vi "Prueba_MAIN.vi"() -> ()   [LabVIEW 2019]
uses:
  Estados_flujo_Debug.ctl
  CLUSTER_CONTROLES_INDICADORES.ctl
  Acciones_UI.ctl
  <vilib>/Instr/_visa.llb/VISA Configure Serial Port (Instr).vi
panel:
  out "Numeric":i32
  in  "Tab Control":enum32{"Page 1", "Page 2"}(tab)
  out "MESSAGES":string
  in  "TEST ASICS":bool
  in  "MOVER ASICS":bool
  in  "LEER QR'S":bool
  in  "CALIBRACION":bool
  in  "Exit":bool
  in  "INICIAR COM":bool
  out "DISPOSITIVO CONECTADO":string
  # "PONER VENTANA DE DIALOGO PARA PREGUNTAR SI SE QUIERE SALIR CUANDO SE PRESIONE STOP"
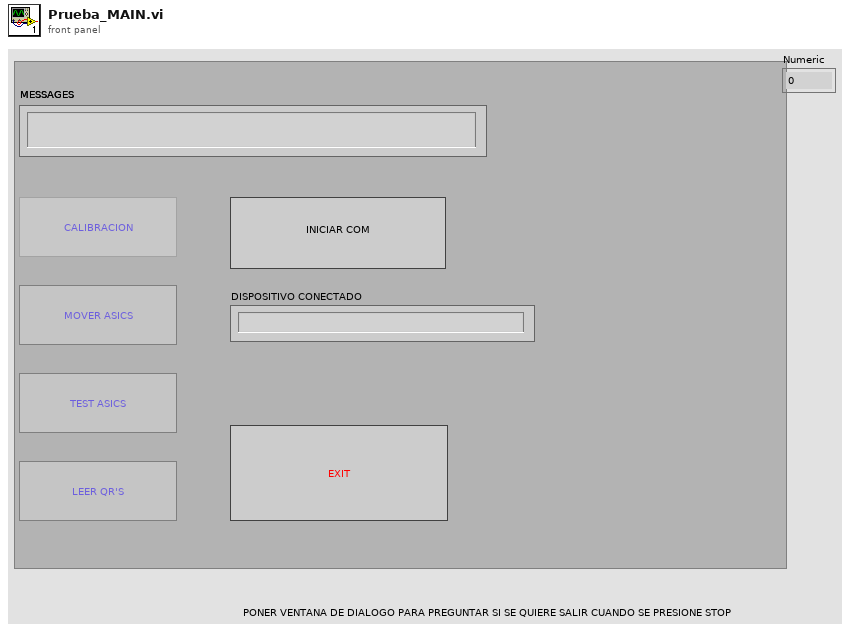
[diagram p1: front panel]
types:
  T1 = typedef "CLUSTER_CONTROLES_INDICADORES.ctl" = cluster{"TEST ASICS":refnum<vi>, "MOVER ASICS":refnum<vi>, "LEER QR'S":refnum<vi>, "MESSAGES":refnum<vi>, "INICIAR COM":refnum<vi>, "stop":refnum<vi>, "CALIBRACION":refnum<vi>}
  T2 = typedef "Estados_flujo_Debug.ctl" = enum16{"Init", "Sesiones Visa abiertas?", "Iniciar Visa", "Start", "Enviar Comando", "Recibir Fin", "Error?"}
  T3 = typedef "Acciones_UI.ctl" = enum16{"Activar", "Desactivar", "Reiniciar default"}
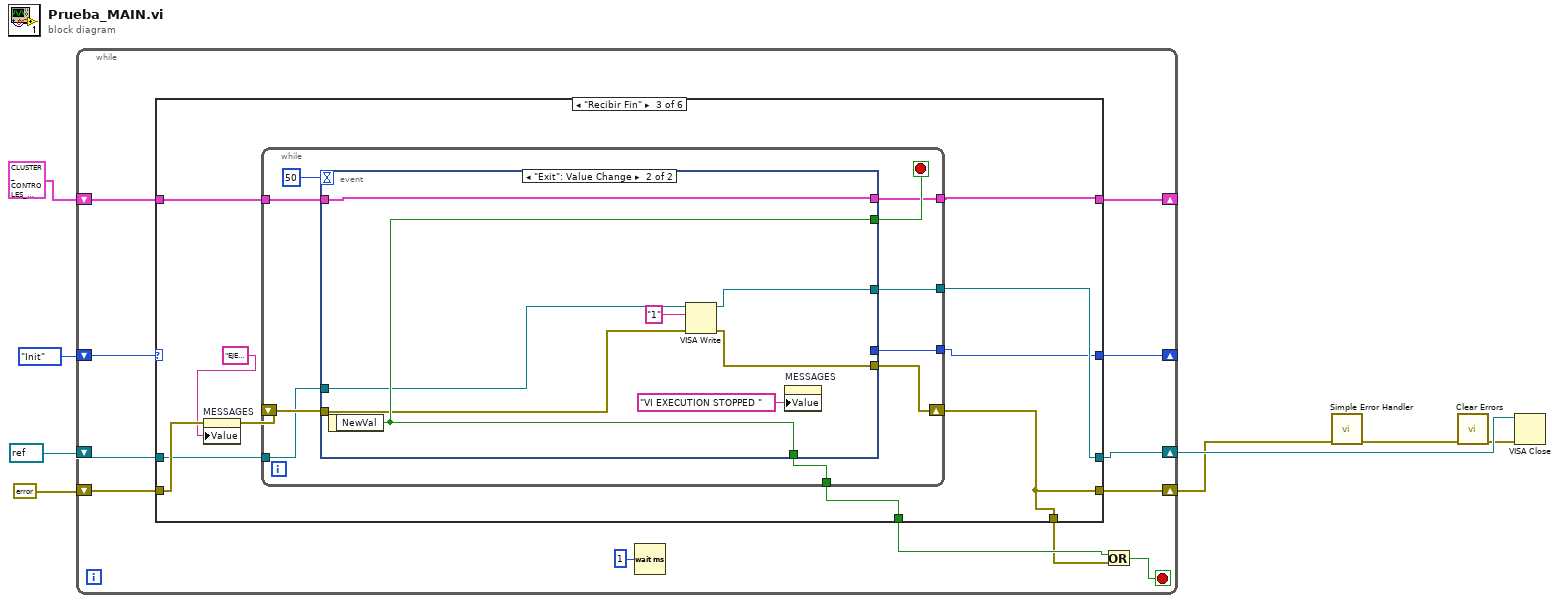
[diagram p0: block diagram]
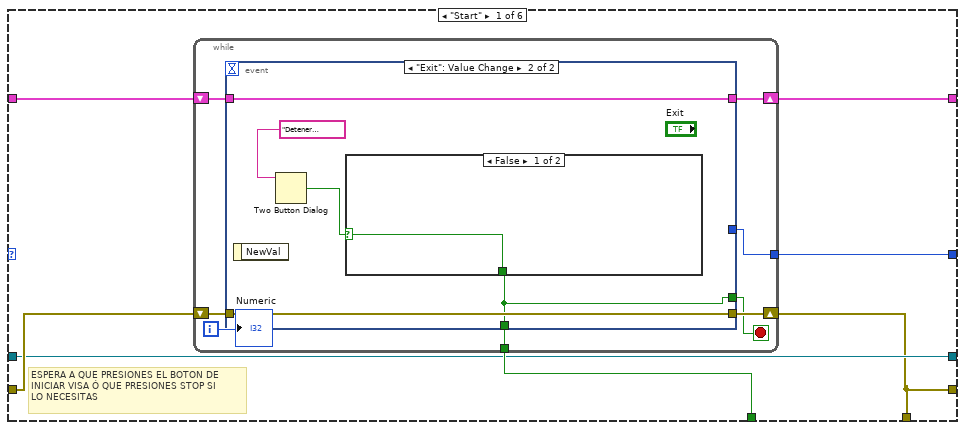
[diagram p2: hidden frame]
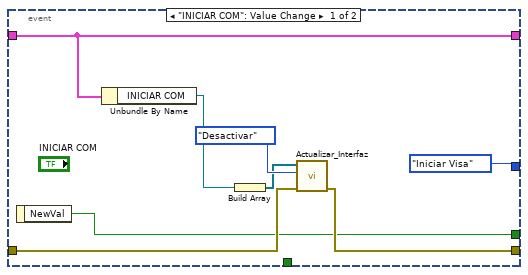
[diagram p3: hidden frame]
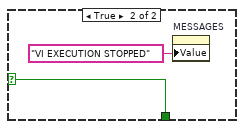
[diagram p4: hidden frame]
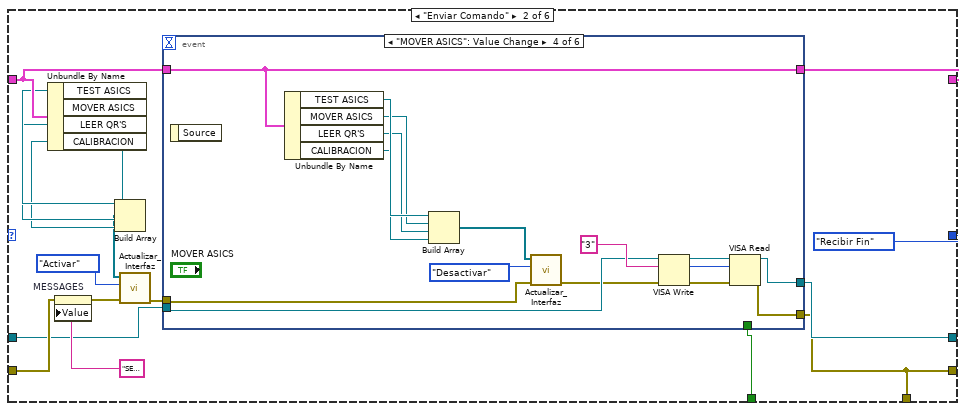
[diagram p5: hidden frame]
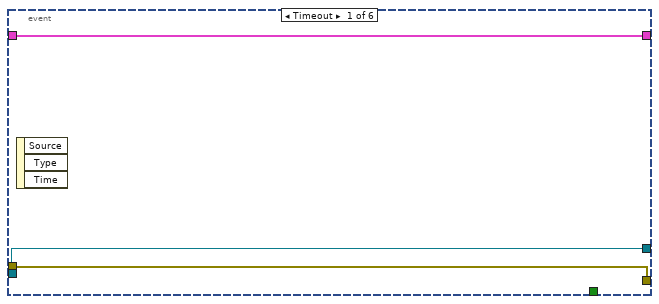
[diagram p6: hidden frame]
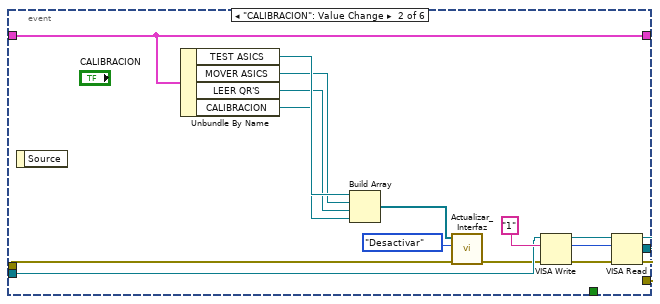
[diagram p7: hidden frame]
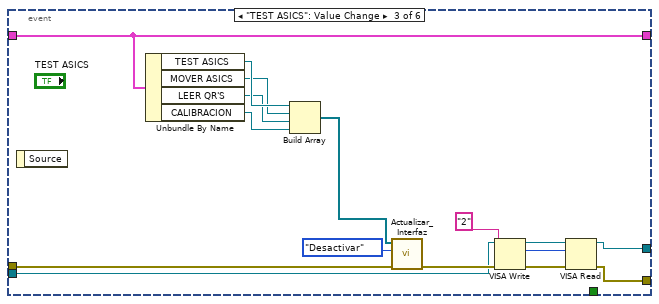
[diagram p8: hidden frame]
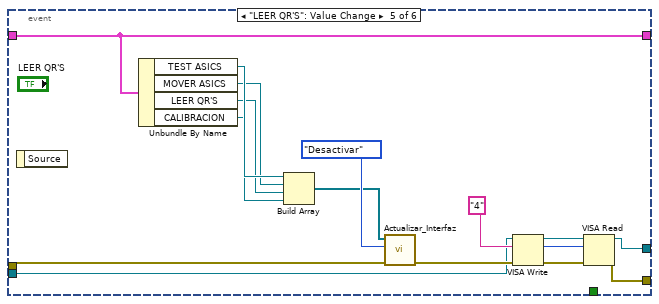
[diagram p9: hidden frame]
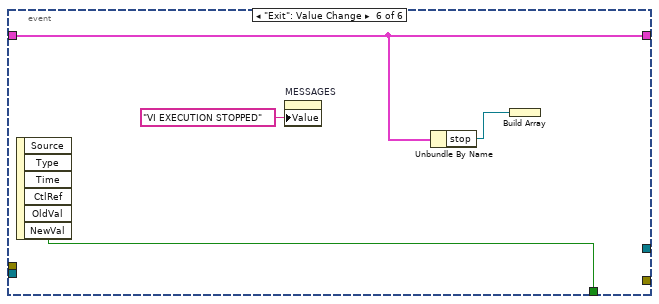
[diagram p10: hidden frame]
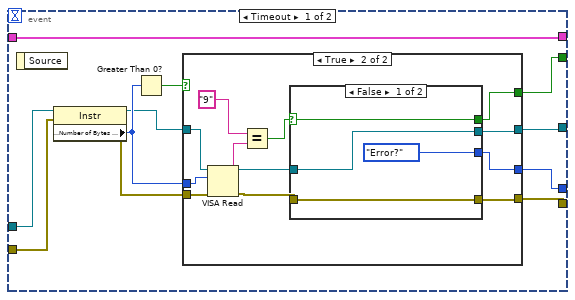
[diagram p11: hidden frame]
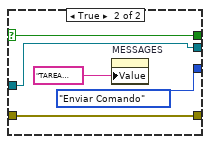
[diagram p13: hidden frame]
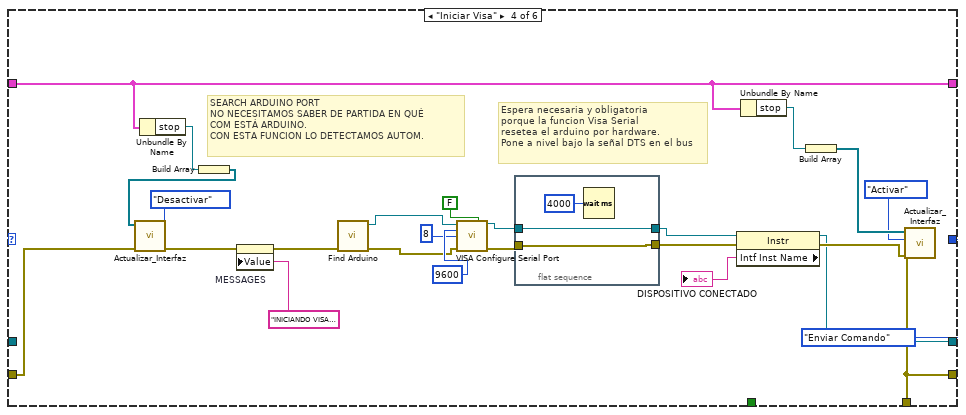
[diagram p14: hidden frame]
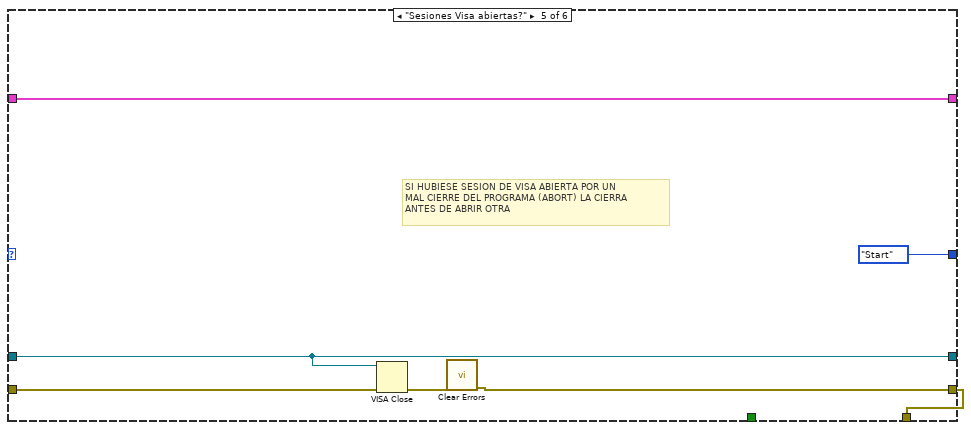
[diagram p15: hidden frame]
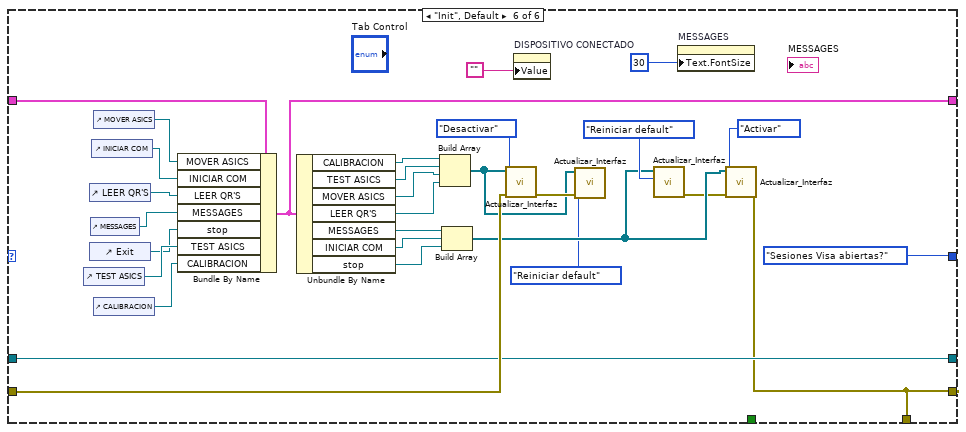
[diagram p16: hidden frame]
diagram:
  n1 = while {
    shift-right: [w17] -> _
    shift-left: Estados_flujo_Debug."Init" -> [w20]
    shift-right: [w16] -> w2
    shift-left: errorcluster {"status"=FALSE, "code"=0, "source"=""} ("error out") -> [w18]
    shift-right: [w10] -> w6
    shift-left: refnum<visa-resource-name> refnum ("VISA resource name out") -> [w11]
    shift-right: [w12] -> _
    shift-left: T1 {"TEST ASICS"=refnum, "MOVER ASICS"=refnum, "LEER QR'S"=refnum, "MESSAGES"=refnum, "INICIAR COM"=refnum, "stop"=refnum, "CALIBRACION"=refnum} ("INDICADORES_CONTROLES") -> [w13]
    stop <- w15 stop-if-true
    n2 = case shown="\"Recibir Fin\"" w20 {
      tunnel: [w27 w68 w143 _ _ _] -> w19
      tunnel: w18 -> [w24 w63 w147 w215 w234 w247]
      tunnel: [w22 w52 w139 w206 w230 w240] -> w16
      tunnel: [w21 Estados_flujo_Debug."Recibir Fin" w138 Estados_flujo_Debug."Enviar Comando" Estados_flujo_Debug."Start" ("f") Estados_flujo_Debug."Sesiones Visa abiertas?"] -> w17
      tunnel: [w23 w65 w144 w201 w231 w245] -> w10
      tunnel: w13 -> [w26 w60 w141 w207 w232 w246]
      tunnel: [w25 w64 w140 w207 w232 w244] -> w12
      tunnel: w11 -> [w23 w62 w142 _ w231 w245]
      tunnel: [w22 w52 w139 w206 w230 w240] -> w9
      frame "Start" {
        # "ESPERA A QUE PRESIONES EL BOTON DE\nINICIAR VISA Ó QUE PRESIONES STOP SI\nLO NECESITAS"
        n3 = while {
          tunnel: [w35] -> w27
          tunnel: [w30] -> w21
          shift-right: [w33] -> w25
          shift-left: w26 -> [w34]
          shift-right: [w31] -> w22
          shift-left: w24 -> [w32]
          i -> [w28]
          stop <- w29 stop-if-true
          n4 = event shown="[1] \"Exit\": Value Change" {
            selector: _ -> [_ _]
            dyn-events: _ -> [_ _]
            timeout: _ -> [_ _]
            tunnel: [_ w44] -> w35
            tunnel: [Estados_flujo_Debug."Iniciar Visa" ("f") _] -> w30
            tunnel: w32 -> [w38 w48]
            tunnel: [w37 w48] -> w31
            tunnel: w34 -> [w41 w46]
            tunnel: [w41 w46] -> w33
            tunnel: [w36 w44] -> w29
            event "INICIAR COM": Value Change {
              n5 = event-data() -> ("NewVal"=w36:bool)  [unwired: 1 in]
              n6 = Unbundle By Name(w41) -> ("INICIAR COM"=w40:refnum<vi>)
              n7 = Build Array(w40) -> (w39:refnum<vi>[])
              n8 = call "Actualizar_Interfaz.vi"("error in (no error)"=w38, "Enum"=Acciones_UI."Desactivar", "Controls"=w39) -> ("error out"=w37:errorcluster)  [unwired: 8 in]
            }
            event "Exit": Value Change {
              n9 = event-data() -> ()  [unwired: 1 in, 1 out]
              n10 = Two Button Dialog(message="Detener ejecución?") -> (T button?=w47:bool)  [unwired: 2 in]
              n11 = case shown="False" w47 {
                selector: w47 -> [w49 w50]
                tunnel: [w49 w50] -> w44
                frame False {
                }
                frame True {
                  n12 = property on="MESSAGES" class="Str"("Value"="VI EXECUTION STOPPED" ("MESSAGES")) -> ()  [unwired: 2 in, 2 out]
                }
              }
            }
          }
          "Numeric" <- w28
        }
      }
      frame "Enviar Comando" {
        n13 = Unbundle By Name(w60) -> ("TEST ASICS"=w59:refnum<vi>, "MOVER ASICS"=w58:refnum<vi>, "LEER QR'S"=w57:refnum<vi>, "CALIBRACION"=w56:refnum<vi>)
        n14 = property on="MESSAGES" class="Str"(error in=w63, "Value"="SELECCIONE TAREA" ("String")) -> (error out=w61:errorcluster)  [unwired: 1 in, 1 out]
        n15 = Build Array(w59, w58, w57, w56) -> (w55:refnum<vi>[])
        n16 = call "Actualizar_Interfaz.vi"("error in (no error)"=w61, "Enum"=Acciones_UI."Activar", "Controls"=w55) -> ("error out"=w66:errorcluster)  [unwired: 8 in]
        n17 = event shown="[3] \"MOVER ASICS\": Value Change" {
          selector: _ -> [_ _ _ _ _ _]
          dyn-events: _ -> [_ _ _ _ _ _]
          timeout: _ -> [_ _ _ _ _ _]
          tunnel: [_ _ _ _ _ w137] -> w68
          tunnel: w66 -> [w69 w73 w95 w104 w127 _]
          tunnel: [w70 w85 w97 w105 w129 _] -> w65
          tunnel: [w69 w84 w98 w114 w128 _] -> w52
          tunnel: w60 -> [w71 w74 w96 w106 w119 w134]
          tunnel: [w71 w74 w96 w106 w119 w134] -> w64
          tunnel: w62 -> [w70 w81 w94 w113 w126 _]
          event Timeout {
            n18 = event-data() -> ()  [unwired: 1 in, 3 out]
          }
          event "CALIBRACION": Value Change {
            n19 = event-data() -> ()  [unwired: 1 in, 1 out]
            n20 = Unbundle By Name(w74) -> ("TEST ASICS"=w80:refnum<vi>, "MOVER ASICS"=w79:refnum<vi>, "LEER QR'S"=w78:refnum<vi>, "CALIBRACION"=w77:refnum<vi>)
            n21 = Build Array(w80, w79, w78, w77) -> (w75:refnum<vi>[])
            n22 = call "Actualizar_Interfaz.vi"("error in (no error)"=w73, "Enum"=Acciones_UI."Desactivar", "Controls"=w75) -> ("error out"=w72:errorcluster)  [unwired: 8 in]
            n23 = VISA Write(VISA resource name=w81, write buffer="1", error in (no error)=w72) -> (VISA resource name out=w86:refnum<visa-resource-name>, return count=w82:u32, error out=w87:errorcluster)
            n24 = VISA Read(VISA resource name=w86, byte count=w82, error in (no error)=w87) -> (VISA resource name out=w85:refnum<visa-resource-name>, error out=w84:errorcluster)  [unwired: 2 out]
          }
          event "TEST ASICS": Value Change {
            n25 = event-data() -> ()  [unwired: 1 in, 1 out]
            n26 = Unbundle By Name(w96) -> ("TEST ASICS"=w93:refnum<vi>, "MOVER ASICS"=w92:refnum<vi>, "LEER QR'S"=w91:refnum<vi>, "CALIBRACION"=w90:refnum<vi>)
            n27 = Build Array(w93, w92, w91, w90) -> (w88:refnum<vi>[])
            n28 = call "Actualizar_Interfaz.vi"("Enum"=Acciones_UI."Desactivar", "Controls"=w88) -> ()  [unwired: 9 in, 1 out]
            n29 = VISA Write(VISA resource name=w94, write buffer="2", error in (no error)=w95) -> (VISA resource name out=w101:refnum<visa-resource-name>, return count=w99:u32, error out=w102:errorcluster)
            n30 = VISA Read(VISA resource name=w101, byte count=w99, error in (no error)=w102) -> (VISA resource name out=w97:refnum<visa-resource-name>, error out=w98:errorcluster)  [unwired: 2 out]
          }
          event "MOVER ASICS": Value Change {
            n31 = event-data() -> ()  [unwired: 1 in, 1 out]
            n32 = Unbundle By Name(w106) -> ("TEST ASICS"=w112:refnum<vi>, "MOVER ASICS"=w111:refnum<vi>, "LEER QR'S"=w110:refnum<vi>, "CALIBRACION"=w109:refnum<vi>)
            n33 = Build Array(w112, w111, w110, w109) -> (w107:refnum<vi>[])
            n34 = call "Actualizar_Interfaz.vi"("error in (no error)"=w104, "Enum"=Acciones_UI."Desactivar", "Controls"=w107) -> ("error out"=w103:errorcluster)  [unwired: 8 in]
            n35 = VISA Write(VISA resource name=w113, write buffer="3", error in (no error)=w103) -> (VISA resource name out=w117:refnum<visa-resource-name>, return count=w115:u32, error out=w118:errorcluster)
            n36 = VISA Read(VISA resource name=w117, byte count=w115, error in (no error)=w118) -> (VISA resource name out=w105:refnum<visa-resource-name>, error out=w114:errorcluster)  [unwired: 2 out]
          }
          event "LEER QR'S": Value Change {
            n37 = event-data() -> ()  [unwired: 1 in, 1 out]
            n38 = Unbundle By Name(w119) -> ("TEST ASICS"=w125:refnum<vi>, "MOVER ASICS"=w124:refnum<vi>, "LEER QR'S"=w123:refnum<vi>, "CALIBRACION"=w122:refnum<vi>)
            n39 = Build Array(w125, w124, w123, w122) -> (w120:refnum<vi>[])
            n40 = call "Actualizar_Interfaz.vi"("Enum"=Acciones_UI."Desactivar", "Controls"=w120) -> ()  [unwired: 9 in, 1 out]
            n41 = VISA Write(VISA resource name=w126, write buffer="4", error in (no error)=w127) -> (VISA resource name out=w132:refnum<visa-resource-name>, return count=w130:u32, error out=w133:errorcluster)
            n42 = VISA Read(VISA resource name=w132, byte count=w130, error in (no error)=w133) -> (VISA resource name out=w129:refnum<visa-resource-name>, error out=w128:errorcluster)  [unwired: 2 out]
          }
          event "Exit": Value Change {
            n43 = event-data() -> ("NewVal"=w137:bool)  [unwired: 1 in, 5 out]
            n44 = property on="MESSAGES" class="Str"("Value"="VI EXECUTION STOPPED" ("MESSAGES")) -> ()  [unwired: 2 in, 2 out]
            n45 = Unbundle By Name(w134) -> ("stop"=w135:refnum<vi>)
            n46 = Build Array(w135) -> ()  [unwired: 1 out]
          }
        }
      }
      frame "Recibir Fin" {
        n47 = property on="MESSAGES" class="Str"(error in=w147, "Value"="EJECUTANDO TAREA" ("String")) -> (error out=w145:errorcluster)  [unwired: 1 in, 1 out]
        n48 = while {
          tunnel: [w155] -> w138
          tunnel: [w153] -> w144
          shift-right: [w152] -> w139
          shift-left: w145 -> [w154]
          tunnel: [w151] -> w143
          tunnel: w142 -> [w150]
          tunnel: w141 -> [w149]
          tunnel: [w148] -> w140
          stop <- w156 stop-if-true
          n49 = event shown="[1] \"Exit\": Value Change" {
            selector: _ -> [_ _]
            dyn-events: _ -> [_ _]
            timeout: 50 -> [_ _]
            tunnel: [w166 w200] -> w156
            tunnel: [w165 _] -> w155
            tunnel: w154 -> [w164 w198]
            tunnel: [w161 w197] -> w152
            tunnel: [w160 w195] -> w153
            tunnel: [_ w200] -> w151
            tunnel: w150 -> [w159 w194]
            tunnel: w149 -> [w158 w193]
            tunnel: [w158 w193] -> w148
            event Timeout {
              n50 = event-data() -> ()  [unwired: 1 in, 1 out]
              n51 = property class="Instr"(reference=w159, error in=w164) -> (reference out=w163:refnum<visa-resource-name>, error out=w162:errorcluster, "Serial Settings:Number of Bytes at Serial Port"=w167:u32)
              n52 = Greater Than 0?(x=w167) -> (x > 0?=w168:bool)
              n53 = case shown="True" w168 {
                selector: w168 -> [w171 _]
                tunnel: w167 -> [_ w183]
                tunnel: [w171 w177] -> w166
                tunnel: [_ w178] -> w165
                tunnel: w163 -> [w170 w180]
                tunnel: w162 -> [w169 w174]
                tunnel: [w169 w172] -> w161
                tunnel: [w170 w176] -> w160
                frame False {
                }
                frame True {
                  n54 = VISA Read(VISA resource name=w180, byte count=w183, error in (no error)=w174) -> (VISA resource name out=w175:refnum<visa-resource-name>, read buffer=w181:string, error out=w173:errorcluster)  [unwired: 1 out]
                  n55 = Equal?(x="9", y=w181) -> (x = y?=w179:bool)
                  n56 = case shown="False" w179 {
                    selector: w179 -> [w186 w190]
                    tunnel: [Estados_flujo_Debug."Error?" Estados_flujo_Debug."Enviar Comando"] -> w178
                    tunnel: [w186 w190] -> w177
                    tunnel: [w185 w189] -> w176
                    tunnel: w175 -> [w185 w189]
                    tunnel: w173 -> [w184 w188]
                    tunnel: [w184 w188] -> w172
                    frame False {
                    }
                    frame True {
                      n57 = property on="MESSAGES" class="Str"("Value"="TAREA TERMINADA" ("String")) -> ()  [unwired: 2 in, 2 out]
                    }
                  }
                }
              }
            }
            event "Exit": Value Change {
              n58 = event-data() -> ("NewVal"=w200:bool)  [unwired: 1 in]
              n59 = VISA Write(VISA resource name=w194, write buffer="1", error in (no error)=w198) -> (VISA resource name out=w195:refnum<visa-resource-name>, error out=w197:errorcluster)  [unwired: 1 out]
              n60 = property on="MESSAGES" class="Str"("Value"="VI EXECUTION STOPPED " ("MESSAGES")) -> ()  [unwired: 2 in, 2 out]
            }
          }
        }
      }
      frame "Iniciar Visa" {
        # "SEARCH ARDUINO PORT\nNO NECESITAMOS SABER DE PARTIDA EN QUÉ\nCOM ESTÁ ARDUINO. \nCON ESTA FUNCION LO DETECTAMOS AUTOM."
        # "Espera necesaria y obligatoria\nporque la funcion Visa Serial\nresetea el arduino por hardware.\nPone a nivel bajo la señal DTS en el bus"
        n61 = Unbundle By Name(w207) -> ("stop"=w213:refnum<vi>)
        n62 = Build Array(w213) -> (w212:refnum<vi>[])
        n63 = call "Actualizar_Interfaz.vi"("error in (no error)"=w215, "Enum"=Acciones_UI."Desactivar", "Controls"=w212) -> ("error out"=w214:errorcluster)  [unwired: 8 in]
        n64 = property on="MESSAGES" class="Str"(error in=w214, "Value"="INICIANDO VISA Y ARDUINO.....ESPERE" ("String")) -> (error out=w218:errorcluster)  [unwired: 1 in, 1 out]
        n65 = call "Find Arduino.vi"("error in (no error)"=w218) -> ("error out"=w223:errorcluster, "VISA resource name"=w222:refnum<visa-resource-name>)  [unwired: 8 in, 1 out]
        n66 = call-poly "VISA Configure Serial Port"("VISA resource name"=w222, "Enable Termination\nChar (T)"=FALSE ("Enable Termination\nChar (T)"), "baud rate (9600)"=u32 9600, "data bits (8)"=u16 8, "error in (no error)"=w223) -> ("VISA resource name out"=w203:refnum<visa-resource-name>, "error out"=w217:errorcluster)  [unwired: 9 in]
        n67 = flat-sequence {
          tunnel: [w227] -> w205
          tunnel: w217 -> [w227]
          tunnel: [w226] -> w202
          tunnel: w203 -> [w226]
          frame #0 {
            n68 = Wait (ms)(milliseconds to wait=u32 4000) -> ()  [unwired: 1 out]
          }
        }
        n69 = property class="Instr"(reference=w202, error in=w205) -> (reference out=w201:refnum<visa-resource-name>, error out=w204:errorcluster, "Intf Inst Name"=→"DISPOSITIVO CONECTADO":string)
        n70 = Unbundle By Name(w207) -> ("stop"=w210:refnum<vi>)
        n71 = Build Array(w210) -> (w209:refnum<vi>[])
        n72 = call "Actualizar_Interfaz.vi"("error in (no error)"=w204, "Enum"=Acciones_UI."Activar", "Controls"=w209) -> ("error out"=w206:errorcluster)  [unwired: 8 in]
      }
      frame "Sesiones Visa abiertas?" {
        # "SI HUBIESE SESION DE VISA ABIERTA POR UN \nMAL CIERRE DEL PROGRAMA (ABORT) LA CIERRA\nANTES DE ABRIR OTRA"
        n73 = VISA Close(VISA resource name=w231, error in (no error)=w234) -> (error out=w233:errorcluster)
        n74 = call <vilib>:"Clear Errors.vi"("error in (no error)"=w233) -> ("error out"=w230:errorcluster)  [unwired: 5 in, 1 out]
      }
      frame "Init", Default {
        n75 = control-ref of="TEST ASICS"() -> (w263:refnum<vi>)
        n76 = control-ref of="LEER QR'S"() -> (w260:refnum<vi>)
        n77 = control-ref of="Exit"() -> (w262:refnum<vi>)
        n78 = control-ref of="MESSAGES"() -> (w261:refnum<vi>)
        n79 = control-ref of="INICIAR COM"() -> (w259:refnum<vi>)
        n80 = control-ref of="MOVER ASICS"() -> (w258:refnum<vi>)
        n81 = control-ref of="CALIBRACION"() -> (w264:refnum<vi>)
        n82 = Bundle By Name(cluster=w246, "MOVER ASICS"=w258, "INICIAR COM"=w259, "LEER QR'S"=w260, "MESSAGES"=w261, "stop"=w262, "TEST ASICS"=w263, "CALIBRACION"=w264) -> (w244:T1)
        n83 = Unbundle By Name(w244) -> ("CALIBRACION"=w254:refnum<vi>, "TEST ASICS"=w253:refnum<vi>, "MOVER ASICS"=w252:refnum<vi>, "LEER QR'S"=w251:refnum<vi>, "MESSAGES"=w250:refnum<vi>, "INICIAR COM"=w249:refnum<vi>, "stop"=w248:refnum<vi>)
        n84 = Build Array(w254, w253, w252, w251) -> (w235:refnum<vi>[])
        n85 = Build Array(w250, w249, w248) -> (w243:refnum<vi>[])
        n86 = call "Actualizar_Interfaz.vi"("error in (no error)"=w247, "Enum"=Acciones_UI."Desactivar", "Controls"=w235) -> ("error out"=w236:errorcluster)  [unwired: 8 in]
        n87 = property on="DISPOSITIVO CONECTADO" class="Str"("Value"="") -> ()  [unwired: 2 in, 2 out]
        n88 = call "Actualizar_Interfaz.vi"("error in (no error)"=w236, "Enum"=Acciones_UI."Reiniciar default", "Controls"=w235) -> ()  [unwired: 8 in, 1 out]
        n89 = call "Actualizar_Interfaz.vi"("Enum"=Acciones_UI."Reiniciar default", "Controls"=w243) -> ("error out"=w241:errorcluster)  [unwired: 9 in]
        n90 = property on="MESSAGES" class="Str"("Text.FontSize"=u32 30 ("Text.Font:Size")) -> ()  [unwired: 2 in, 2 out]
        n91 = call "Actualizar_Interfaz.vi"("error in (no error)"=w241, "Enum"=Acciones_UI."Activar", "Controls"=w243) -> ("error out"=w240:errorcluster)  [unwired: 8 in]
      }
    }
    n92 = Wait (ms)(milliseconds to wait=u32 1) -> ()  [unwired: 1 out]
    n93 = Or(x=w19, y=w9) -> (x .or. y?=w15:bool)
  }
  n94 = call <vilib>:"Simple Error Handler.vi"("error in (no error)"=w2) -> ("error out"=w1:errorcluster)  [unwired: 4 in, 4 out]
  n95 = call <vilib>:"Clear Errors.vi"("error in (no error)"=w1) -> ("error out"=w5:errorcluster)  [unwired: 5 in, 1 out]
  n96 = VISA Close(VISA resource name=w6, error in (no error)=w5) -> ()  [unwired: 1 out]
